vi "Muted.vi"(8 "error in (no error)":errorcluster, 11 "RGetInputMute in":refnum<class "RGetInputMute.lvclass">) -> (0 "error out":errorcluster, 2 "Muted":bool, 3 "RGetInputMute out":refnum<class "RGetInputMute.lvclass">)   [LabVIEW 2022 SP3, in "obs-websocket-lv.lvlib" / "RGetInputMute.lvclass"]
uses:
  RGetInputMute.lvclass
  RGetInputMute.lvclass/RGetInputMute.ctl
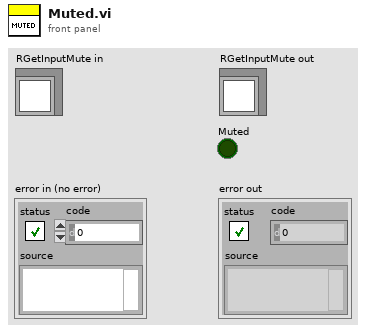
[diagram p1: front panel]
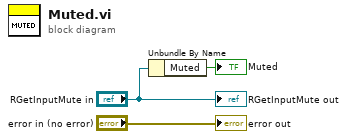
[diagram p0: block diagram]
diagram:
  n1 = Unbundle By Name("RGetInputMute in") -> ("Muted"=→"Muted":bool)
  "error out" <- "error in (no error)"
  "RGetInputMute out" <- "RGetInputMute in"
